vi "Edit Paths in XML File.vi"(8 "error in":errorcluster, 11 "custom device path":path=path "C:/Users/nitest/Documents/LabVIEW Data") -> (0 "error out":errorcluster, 3 "custom device path out":path=path "C:/Users/nitest/Documents/LabVIEW Data")   [LabVIEW 2020, in "Template Tool.lvlib"]
uses:
  Template Tool.lvlib
  Template Tool Global.vi
panel:
  out "number of replacements":i32
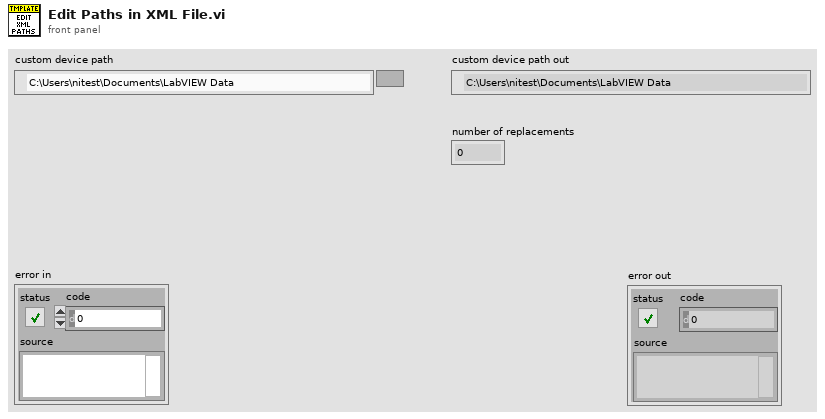
[diagram p1: front panel]
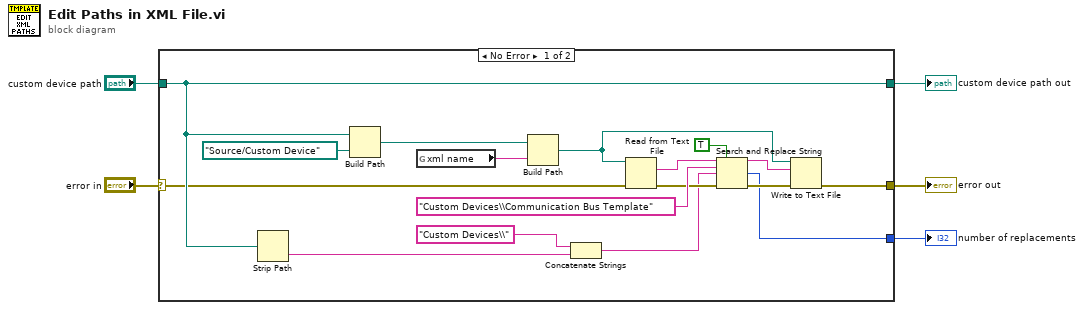
[diagram p0: block diagram]
diagram:
  n1 = case shown="No Error" "error in" {
    selector: "error in" -> [w7 w23]
    tunnel: "custom device path" -> [w8 w24]
    tunnel: [w17 w23] -> w4
    tunnel: [w15 _] -> w3
    tunnel: [w8 w24] -> w2
    frame No Error {
      n2 = Strip Path(path=w8) -> (name=w11:string)  [unwired: 1 out]
      n3 = Build Path(base path=w8, name or relative path=path "Source/Custom Device") -> (appended path=w10:path)
      n4 = global read "Template Tool Global.vi" "xml name"() -> (w6:string)
      n5 = Build Path(base path=w10, name or relative path=w6) -> (appended path=w9:path)
      n6 = Concatenate Strings("Custom Devices\\" ("string"), w11) -> (w12:string)
      n7 = Read from Text File(file (use dialog)=w9, error in=w7) -> (text=w21:string, error out=w19:errorcluster)  [unwired: 2 in, 2 out]
      n8 = Search and Replace String(replace all?=TRUE ("replace all? (F)"), input string=w21, search string="Custom Devices\\Communication Bus Template" ("string"), replace string=w12, error in=w19) -> (result string=w16:string, number of replacements=w15:i32, error out=w18:errorcluster)  [unwired: 3 in, 1 out]
      n9 = Write to Text File(file (use dialog)=w9, text=w16, error in=w18) -> (error out=w17:errorcluster)  [unwired: 1 in, 2 out]
    }
    frame Error {
    }
  }
  "error out" <- w4
  "custom device path out" <- w2
  "number of replacements" <- w3
